vi "GraphSubVi.vi"(2 "reference out":refnum<vi>, 3 "Phase Data":dbl=1.0 min=0.0 max=360.0 step=1.0, 4 "Waveform Type":T1(ring), 5 "Frequency Data":dbl min=1.0 max=37500000.0 step=1.0 format="%#_10g") -> (1 "Waveform Graph":dynamicdata(graph))   [LabVIEW 2024]
panel:
  out "Waveform Graph 2":dynamicdata(graph)
  out "x*y":dbl
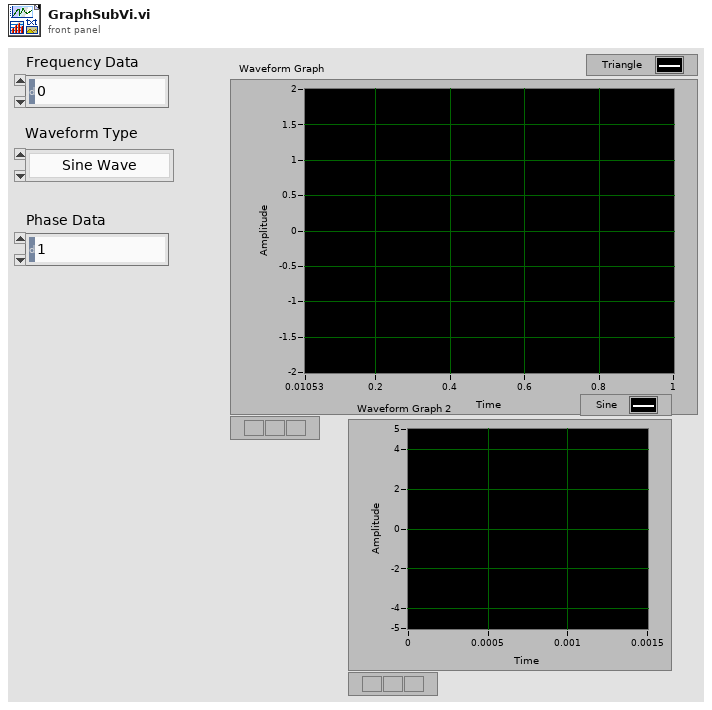
[diagram p1: front panel]
types:
  T1 = enum16{"Sine Wave", "Triangular Wave", "Square Wave"}
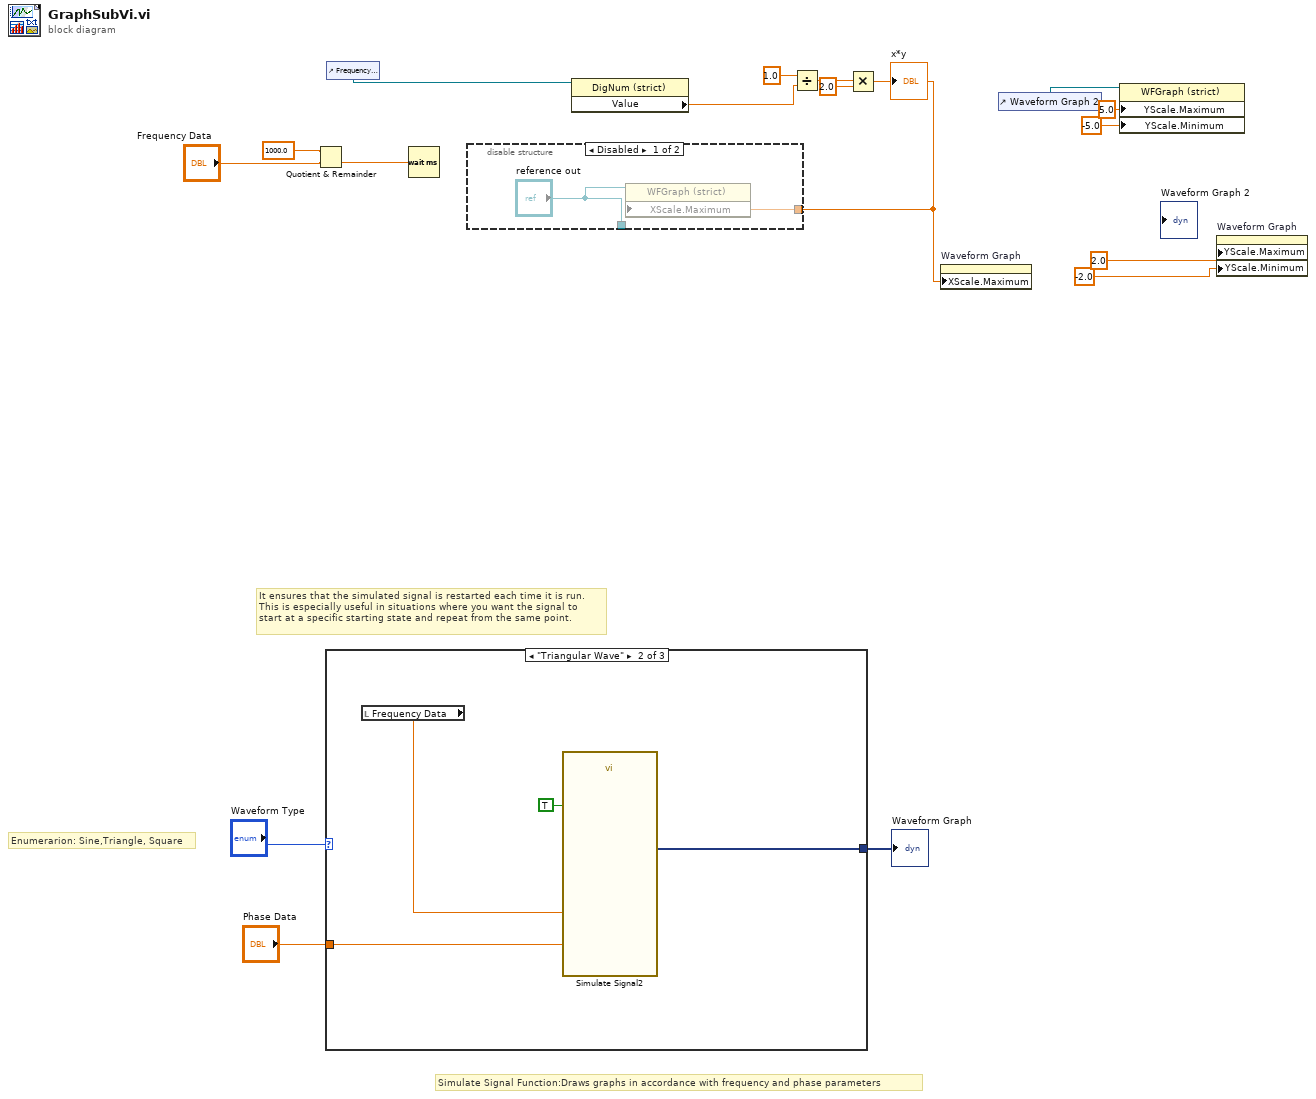
[diagram p0: block diagram]
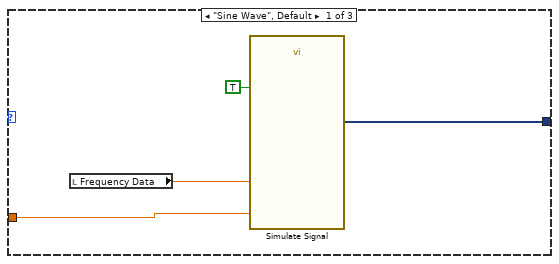
[diagram p3: hidden frame]
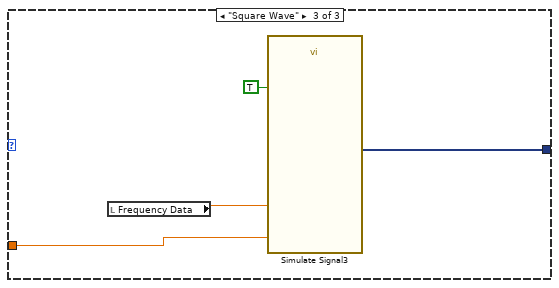
[diagram p4: hidden frame]
diagram:
  # "It ensures that the simulated signal is restarted each time it is run. \nThis is especially useful in situations where you want the signal to \nstart at a specific starting state and repeat from the same point."
  # "Simulate Signal Function:Draws graphs in accordance with frequency and phase parameters"
  # "Enumerarion: Sine,Triangle, Square"
  n1 = Quotient & Remainder(x=1000.0, y="Frequency Data") -> (floor(x/y)=w7:dbl)  [unwired: 1 out]
  n2 = case shown="\"Triangular Wave\"" "Waveform Type" {
    tunnel: [w20 w25 w29] -> w6
    tunnel: "Phase Data" -> [w19 w24 w27]
    frame "Sine Wave", Default {
      n3 = local read "Frequency Data"() -> (w21:dbl)
      n4 = call "Simulate Signal"("Reset Signal"=TRUE, "Frequency"=w21, "Phase"=w19) -> ("Sine"=w20:dynamicdata)  [unwired: 11 in, 1 out]
    }
    frame "Triangular Wave" {
      n5 = local read "Frequency Data"() -> (w23:dbl)
      n6 = call "Simulate Signal2"("Reset Signal"=TRUE, "Frequency"=w23, "Phase"=w24) -> ("Triangle"=w25:dynamicdata)  [unwired: 11 in, 1 out]
    }
    frame "Square Wave" {
      n7 = local read "Frequency Data"() -> (w28:dbl)
      n8 = call "Simulate Signal3"("Reset Signal"=TRUE, "Frequency"=w28, "Phase"=w27) -> ("Square"=w29:dynamicdata)  [unwired: 11 in, 1 out]
    }
  }
  "Waveform Graph" <- w6
  n9 = control-ref of="Frequency Data"() -> (w11:refnum<vi>)
  n10 = Wait (ms)(milliseconds to wait=w7) -> ()  [unwired: 1 out]
  n11 = property class="DigNum (strict)"(reference=w11) -> ("Value"=w10:dbl)  [unwired: 1 in, 2 out]
  n12 = Divide(x=1.0, y=w10) -> (x/y=w14:dbl)
  n13 = Multiply(x=w14, y=2.0) -> (x*y=w9:dbl)
  "x*y" <- w9
  n14 = disable-structure shown="Disabled" {
    disable-tunnel: w9 -> [w31 _]
    disable-tunnel: ["reference out" _] -> _
    frame Disabled {
      n15 = property class="WFGraph (strict)"(reference="reference out", "XScale.Maximum"=w31) -> ()  [unwired: 1 in, 2 out]
    }
    frame Enabled {
    }
  }
  n16 = property on="Waveform Graph" class="WFGraph (strict)"("XScale.Maximum"=w9) -> ()  [unwired: 2 in, 2 out]
  n17 = control-ref of="Waveform Graph 2"() -> (w3:refnum<vi>)
  n18 = property class="WFGraph (strict)"(reference=w3, "YScale.Maximum"=5.0 ("Y Scale.Range:Maximum"), "YScale.Minimum"=-5.0 ("Y Scale.Range:Minimum")) -> ()  [unwired: 1 in, 2 out]
  n19 = property on="Waveform Graph" class="WFGraph (strict)"("YScale.Maximum"=2.0 ("Y Scale.Range:Maximum"), "YScale.Minimum"=-2.0 ("Y Scale.Range:Minimum")) -> ()  [unwired: 2 in, 2 out]
